vi "CalculateAxis.vi"(8 "error in (no error)":errorcluster, 10 "AcqID":i32, 11 "Automation Refnum in":refnum<k7>) -> (0 "error out":errorcluster, 3 "Spectrum":T1)   [LabVIEW 2014]
uses:
  Spectral Data.ctl
  GetValue Mode.ctl
panel:
  # "LICENSED MATERIALS – PROPERTY OF IBM\nCopyright IBM Corp. 2016,\nALL RIGHTS RESERVED"
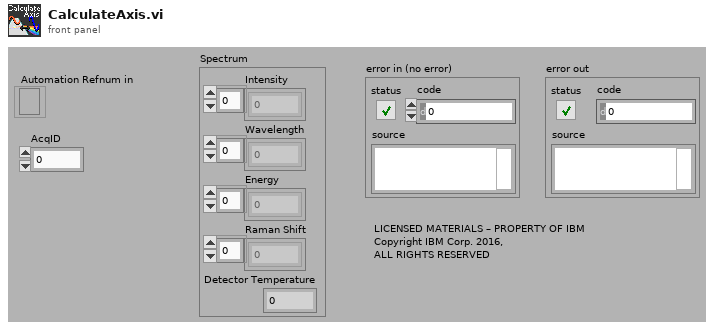
[diagram p1: front panel]
types:
  T1 = typedef "Spectral Data.ctl" = cluster{"Intensity":dbl[], "Wavelength":dbl[], "Energy":dbl[], "Raman Shift":dbl[], "Detector Temperature":dbl}
  T2 = typedef "GetValue Mode.ctl" = enum16{"XY Data", "Data", "MapPoint: Spectrum Index", "Axis Labels", "Axis Units", "Axis", "Axis Index", "Axis Size", "Axis Type", "Intensity", "Frequency", "X", "Y", "Z", "Time", "Double Cursor", "Pointer Limits", "Active Cursors", "Nearest Axis Index", "Acquisition Information", "Custom Information", "History Information", "Data Name", "Dispersion", "Dispersion Parameters", "Labspec Path", "User Level", "System Name", "Autofocus Diode", "Exposure Time", "Live Time", "Labspec Accumulation", "Alignment Diode"}
  T3 = enum16{"cm-1 -> nm", "nm -> cm-1", "eV -> nm", "nm -> eV"}
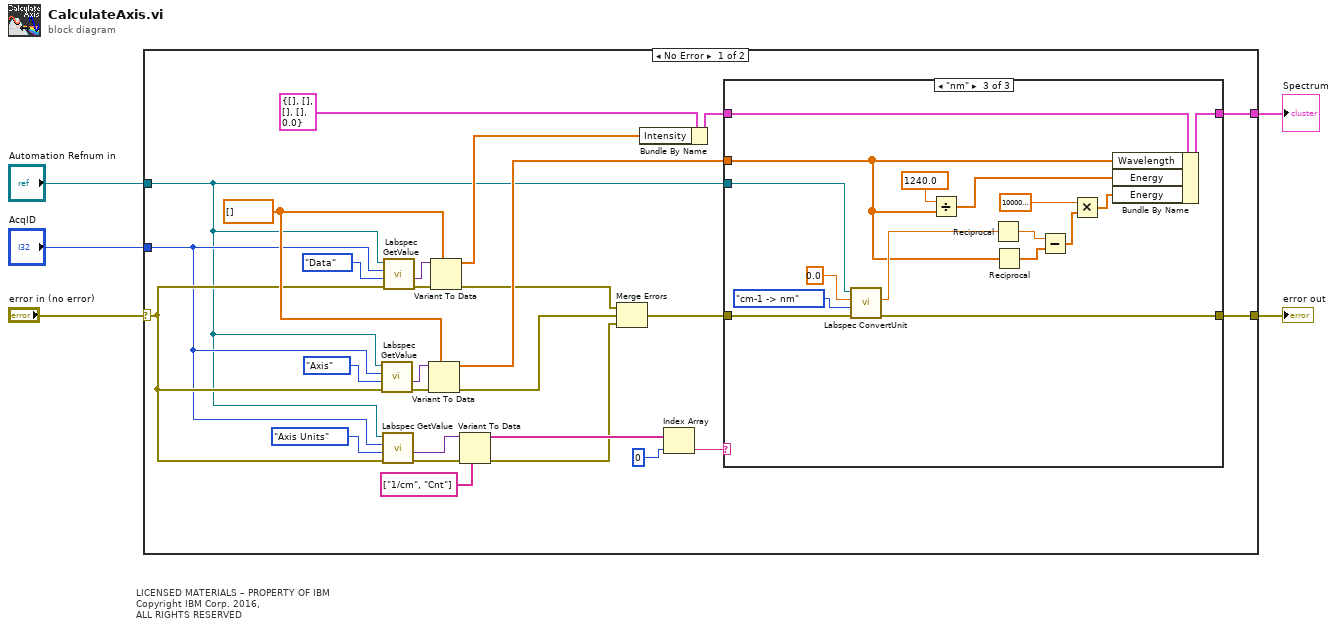
[diagram p0: block diagram]
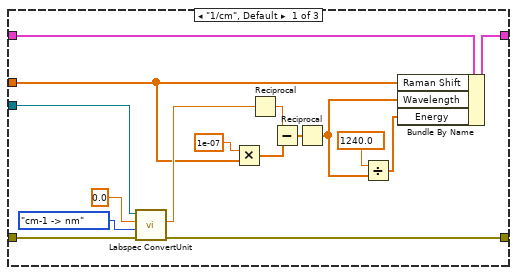
[diagram p2: hidden frame]
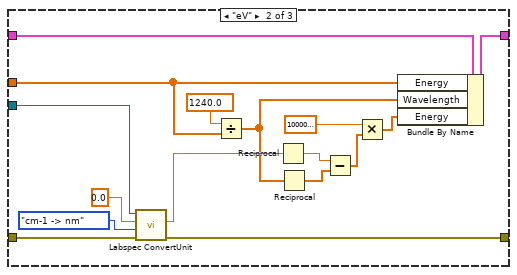
[diagram p3: hidden frame]
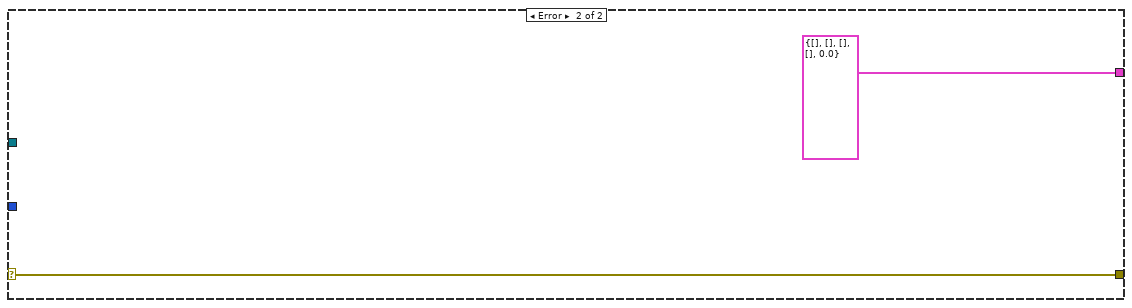
[diagram p4: hidden frame]
diagram:
  # "LICENSED MATERIALS – PROPERTY OF IBM\nCopyright IBM Corp. 2016,\nALL RIGHTS RESERVED"
  n1 = case shown="No Error" "error in (no error)" {
    selector: "error in (no error)" -> [w8 w81]
    tunnel: [w25 w81] -> w5
    tunnel: [w26 T1 {"Intensity"=[], "Wavelength"=[], "Energy"=[], "Raman Shift"=[], "Detector Temperature"=0.0} ("Spectrum")] -> w4
    tunnel: "Automation Refnum in" -> [w6 _]
    tunnel: "AcqID" -> [w7 _]
    frame No Error {
      w20 = dbl[] [] ("data")
      n2 = call "Labspec GetValue.vi"("error in"=w8, "GetValue Mode"=GetValue_Mode."Axis" ("Acquisition Mode"), "DataID"=w7, "Automation Refnum In"=w6) -> ("error out"=w16:errorcluster, "pValue"=w18:variant)  [unwired: 1 in, 5 out]
      n3 = call "Labspec GetValue.vi"("error in"=w8, "GetValue Mode"=GetValue_Mode."Axis Units", "DataID"=w7, "Automation Refnum In"=w6) -> ("error out"=w10:errorcluster, "pValue"=w11:variant)  [unwired: 1 in, 5 out]
      n4 = call "Labspec GetValue.vi"("error in"=w8, "GetValue Mode"=GetValue_Mode."Data" ("Acquisition Mode"), "DataID"=w7, "Automation Refnum In"=w6) -> ("error out"=w13:errorcluster, "pValue"=w15:variant)  [unwired: 1 in, 5 out]
      n5 = Variant To Data(error in=w16, type=w20, Variant=w18) -> (data=w28:dbl[], error out=w22:errorcluster)
      n6 = Variant To Data(error in=w13, type=w20, Variant=w15) -> (data=w19:dbl[], error out=w21:errorcluster)
      n7 = Variant To Data(error in=w10, type=string[] ["1/cm", "Cnt"] ("Array 2"), Variant=w11) -> (data=w32:string[], error out=w24:errorcluster)
      n8 = Merge Errors(w21, w22, w24) -> (w23:errorcluster)
      n9 = Bundle By Name(cluster=T1 {"Intensity"=[], "Wavelength"=[], "Energy"=[], "Raman Shift"=[], "Detector Temperature"=0.0} ("Spectrum"), "Intensity"=w19) -> (w27:T1)
      n10 = Index Array(array=w32, index=0) -> (element=w29:string)
      n11 = case shown="\"nm\"" w29 {
        tunnel: w28 -> [w39 w56 w66]
        tunnel: w27 -> [w48 w64 w80]
        tunnel: [w47 w63 w79] -> w26
        tunnel: [w46 w62 w78] -> w25
        tunnel: w6 -> [w45 w61 w77]
        tunnel: w23 -> [w33 w49 w65]
        frame "1/cm", Default {
          n12 = call "Labspec ConvertUnit.vi"("error in"=w33, "Direction"=T3."cm-1 -> nm", "Initial Value"=0.0, "Automation Refnum In"=w45) -> ("error out"=w46:errorcluster, "Converted Value"=w41:dbl)  [unwired: 5 in, 1 out]
          n13 = Multiply(x=1e-07, y=w39) -> (x*y=w38:dbl[])
          n14 = Reciprocal(x=w41) -> (1/x=w40:dbl)
          n15 = Subtract(x=w40, y=w38) -> (x-y=w42:dbl[])
          n16 = Reciprocal(x=w42) -> (1/x=w35:dbl[])
          n17 = Divide(x=1240.0, y=w35) -> (x/y=w34:dbl[])
          n18 = Bundle By Name(cluster=w48, "Raman Shift"=w39, "Wavelength"=w35, "Energy"=w34) -> (w47:T1)
        }
        frame "eV" {
          n19 = call "Labspec ConvertUnit.vi"("error in"=w49, "Direction"=T3."cm-1 -> nm", "Initial Value"=0.0, "Automation Refnum In"=w61) -> ("error out"=w62:errorcluster, "Converted Value"=w58:dbl)  [unwired: 5 in, 1 out]
          n20 = Divide(x=1240.0, y=w56) -> (x/y=w51:dbl[])
          n21 = Reciprocal(x=w58) -> (1/x=w53:dbl)
          n22 = Reciprocal(x=w51) -> (1/x=w52:dbl[])
          n23 = Subtract(x=w53, y=w52) -> (x-y=w54:dbl[])
          n24 = Multiply(x=10000000.0, y=w54) -> (x*y=w50:dbl[])
          n25 = Bundle By Name(cluster=w64, "Energy"=w56, "Wavelength"=w51, "Energy"=w50) -> (w63:T1)
        }
        frame "nm" {
          n26 = call "Labspec ConvertUnit.vi"("error in"=w65, "Direction"=T3."cm-1 -> nm", "Initial Value"=0.0, "Automation Refnum In"=w77) -> ("error out"=w78:errorcluster, "Converted Value"=w74:dbl)  [unwired: 5 in, 1 out]
          n27 = Divide(x=1240.0, y=w66) -> (x/y=w68:dbl[])
          n28 = Reciprocal(x=w74) -> (1/x=w70:dbl)
          n29 = Reciprocal(x=w66) -> (1/x=w69:dbl[])
          n30 = Subtract(x=w70, y=w69) -> (x-y=w71:dbl[])
          n31 = Multiply(x=10000000.0, y=w71) -> (x*y=w67:dbl[])
          n32 = Bundle By Name(cluster=w80, "Wavelength"=w66, "Energy"=w68, "Energy"=w67) -> (w79:T1)
        }
      }
    }
    frame Error {
    }
  }
  "error out" <- w5
  "Spectrum" <- w4
